vi "Process File.vi"(8 "error in (no error)":errorcluster, 10 "File":path, 11 "Line Detector in":refnum<class "Line Detector.lvclass">) -> (0 "error out":errorcluster, 2 "File out":path, 3 "Line Detector out":refnum<class "Line Detector.lvclass">)   [LabVIEW 2016, in "Line Detector.lvclass"]
uses:
  Line Detector.lvclass
  Measure_core/Process Object/Process Object.lvclass
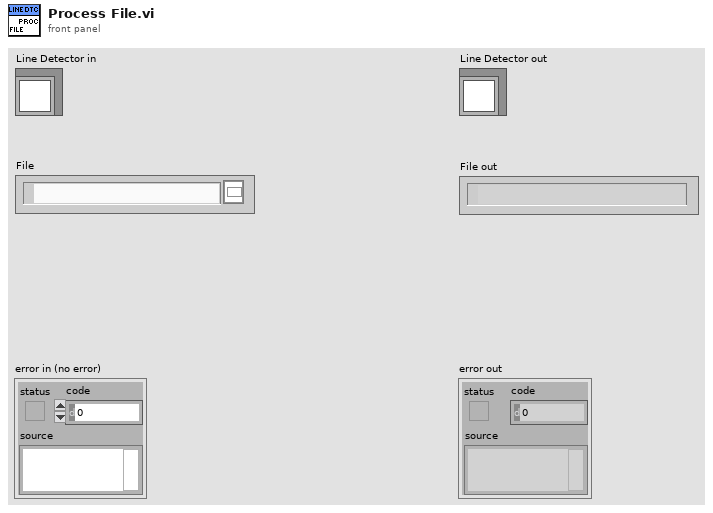
[diagram p1: front panel]
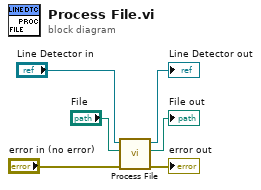
[diagram p0: block diagram]
diagram:
  n1 = call-parent "Process File.vi"("error in (no error)"="error in (no error)", "File"="File", "Process Object in"="Line Detector in") -> ("error out"=→"error out":errorcluster, "File out"=→"File out":path, "Process Object out"=→"Line Detector out":refnum<class "Line Detector.lvclass">)  [unwired: 6 in]
